vi "setUp.vi"(8 "error in (no error)":errorcluster, 11 "reference in":refnum<class "SLSC Switch ActionVIOnCompile Unit Tests.lvclass">) -> (0 "error out":errorcluster, 3 "reference out":refnum<class "SLSC Switch ActionVIOnCompile Unit Tests.lvclass">)   [LabVIEW 2017, in "SLSC Switch ActionVIOnCompile Unit Tests.lvclass"]
doc: "setUp runs prior to the test method during test execution. Use this method to initialize any object data required by your tests."
uses:
  SLSC Switch ActionVIOnCompile Unit Tests.lvclass
  C:/Program Files (x86)/National Instruments/LabVIEW 2017/vi.lib/addons/_JKI Toolkits/VI Tester/TestCase.llb/TestCase.lvclass
  NationalInstruments.VeriStand.SystemDefinitionAPI
  SLSC Switch ActionVIOnCompile Unit Tests.lvclass/SLSC Switch ActionVIOnCompile Unit Tests.ctl
  <userlib>/_OpenG.lib/file/file.llb/Append Path to Root if Relative - Scalar__ogtk.vi
  <vilib>/addons/_JKI Toolkits/VI Tester/TestCase.llb/TestCase.lvclass
  niveristand-custom-device-testing-tools/VeriStandTestUtilities/VeriStandTestUtilities.lvlib
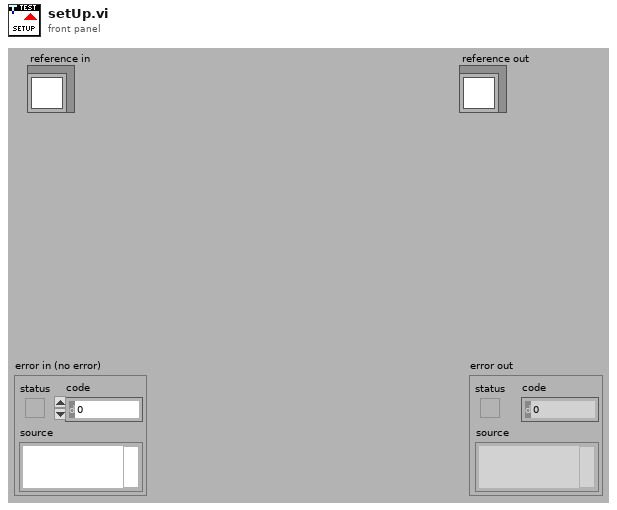
[diagram p1: front panel]
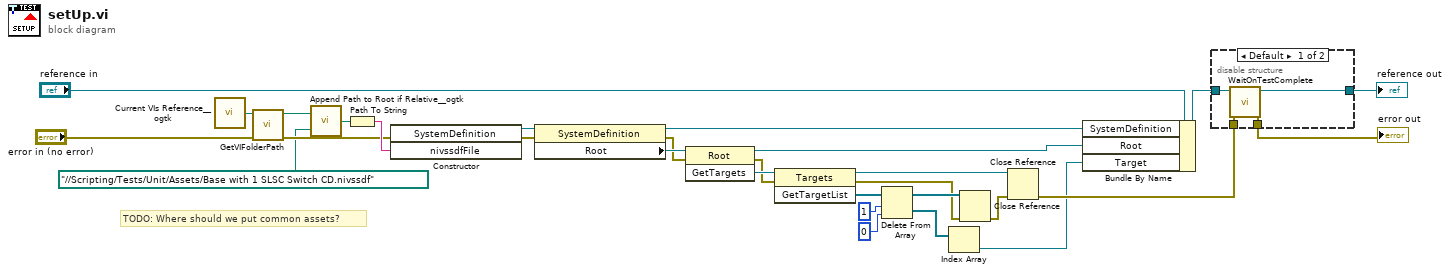
[diagram p0: block diagram]
diagram:
  # "TODO: Where should we put common assets?"
  n1 = call <userlib>:"Current VIs Reference__ogtk.vi"() -> ("Current VI's reference"=w11:refnum<vi>)  [unwired: 5 in]
  n2 = call "GetVIFolderPath.vi"("error in (no error)"="error in (no error)", "VI Reference in"=w11) -> ("error out"=w14:errorcluster, "VI Folder Path out"=w12:path)  [unwired: 8 in]
  n3 = call-poly <userlib>:"Append Path to Root if Relative__ogtk.vi"("Absolute or Relative Path"=path "../../Scripting/Tests/Unit/Assets/Base with 1 SLSC Switch CD.nivssdf", "Root Path"=w12) -> ("Absolute or Appended Path"=w13:path)
  n4 = Path To String(path=w13) -> (string=w16:string)
  n5 = constructor class="SystemDefinition"(error in=w14, "nivssdfFile"=w16) -> (reference out=w17:refnum<k24>, error out=w15:errorcluster)  [unwired: 2 in, 2 out]
  n6 = property class="SystemDefinition"(reference=w17, error in=w15) -> (reference out=w3:refnum<k24>, error out=w18:errorcluster, "Root"=w19:refnum<k24>)
  n7 = invoke class="Root" method="GetTargets"(reference=w19, error in=w18) -> (reference out=w2:refnum<k24>, error out=w20:errorcluster, "GetTargets"=w21:refnum<k24>)  [unwired: 1 in]
  n8 = invoke class="Targets" method="GetTargetList"(reference=w21, error in=w20) -> (reference out=w26:refnum<k24>, error out=w23:errorcluster, "GetTargetList"=w22:refnum<k24>[])  [unwired: 1 in]
  n9 = Delete From Array(array=w22, length=1, index=0) -> (deleted portion=w27:refnum<k24>[], array with subset deleted=w24:refnum<k24>[])
  n10 = Index Array(array=w27) -> (element=w1:refnum<k24>)  [unwired: 1 in]
  n11 = Close Reference(reference=w24, error in (no error)=w23) -> (error out=w25:errorcluster)
  n12 = Close Reference(reference=w26, error in (no error)=w25) -> (error out=w6:errorcluster)
  n13 = Bundle By Name(cluster="reference in", "SystemDefinition"=w3, "Root"=w2, "Target"=w1) -> (w4:refnum<class "SLSC Switch ActionVIOnCompile Unit Tests.lvclass">)
  n14 = disable-structure shown="Default" {
    disable-tunnel: w6 -> [w33 w34]
    disable-tunnel: [w32 w34] -> w29
    disable-tunnel: [w31 w35] -> w28
    disable-tunnel: w4 -> [w30 w35]
    frame condition #0 (active) {
      n15 = call <vilib>:"WaitOnTestComplete.vi"("error in (no error)"=w33, "TestCase in"=w30) -> ("error out"=w32:errorcluster, "TestCase out"=w31:refnum<class "SLSC Switch ActionVIOnCompile Unit Tests.lvclass">)  [unwired: 8 in]
    }
    frame condition #1 {
    }
  }
  "error out" <- w29
  "reference out" <- w28
